vi "GetType.vi"(0 "reference in":refnum<class "ValveModbus.lvclass">, 11 "error in (no error)":errorcluster) -> (4 "reference out":refnum<class "ValveModbus.lvclass">, 6 "obj_type":T1, 15 "error out":errorcluster)   [LabVIEW 2019, in "ValveModbus.lvclass"]
uses:
  ValveModbus.lvclass
  Logger_class/ObjType.ctl
  Logger_class/Logger.lvclass
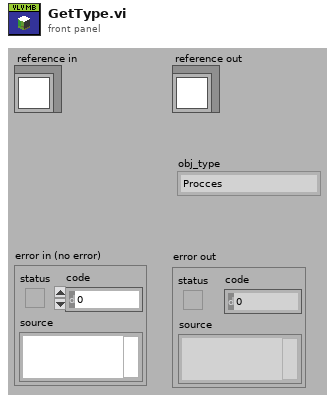
[diagram p1: front panel]
types:
  T1 = typedef "Logger.lvclass/ObjType.ctl" = enum16{"Procces", "Device", "SignalA", "SignalD", "DI", "DO", "DA", "AI", "AO", "AA", "GUI"}
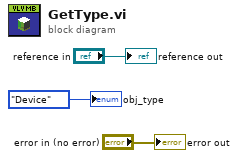
[diagram p0: block diagram]
diagram:
  "error out" <- "error in (no error)"
  "reference out" <- "reference in"
  "obj_type" <- ObjType."Device" ("obj_type")
